vi "MoveRel.vi"(0 "ASI stage":T1, 1 "Axis configuration":u16(ring)=5 items=["No axis", "X", "Y", "Z", "XY", "XYZ"], 5 "x":dbl, 7 "y":dbl, 9 "z":dbl, 11 "error in (no error)":errorcluster) -> (4 "ASI stage out":T1, 15 "error out":errorcluster)   [LabVIEW 2010]
uses:
  stage properties.ctl
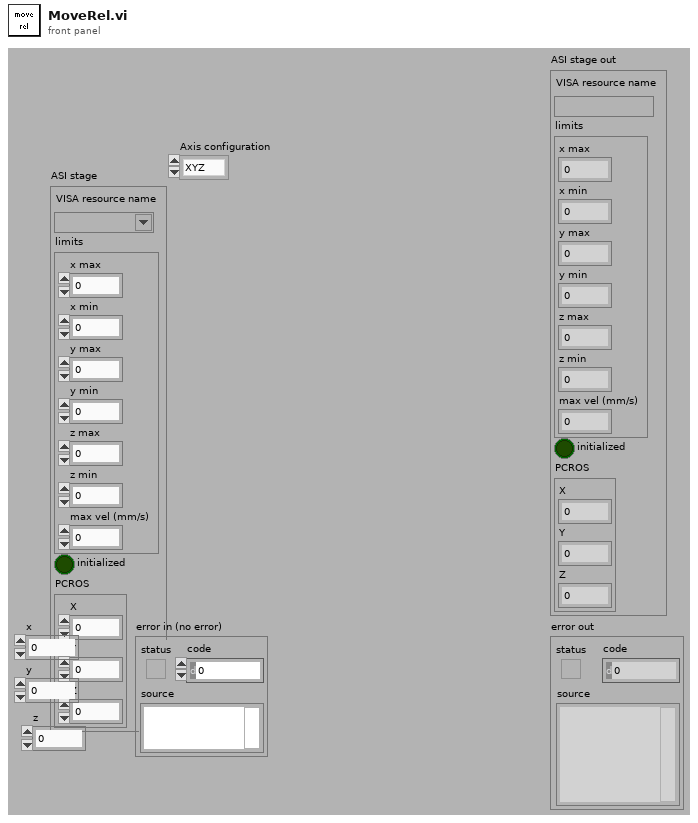
[diagram p1: front panel]
types:
  T1 = typedef "stage properties.ctl" = cluster{"VISA resource name":refnum<visa-resource-name>, "limits":cluster{"x max":dbl, "x min":dbl, "y max":dbl, "y min":dbl, "z max":dbl, "z min":dbl, "max vel (mm/s)":dbl}, "initialized":bool, "PCROS":cluster{"X":dbl, "Y":dbl, "Z":dbl}}
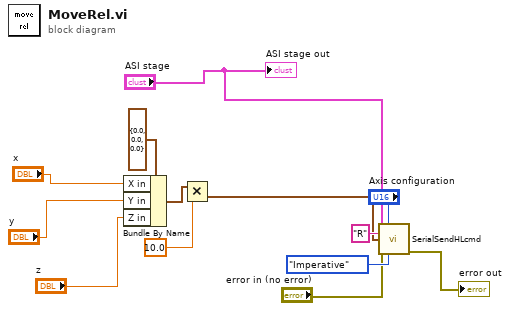
[diagram p0: block diagram]
diagram:
  n1 = Bundle By Name(cluster=cluster{"X in":dbl, "Y in":dbl, "Z in":dbl} {"X in"=0.0, "Y in"=0.0, "Z in"=0.0} ("data in"), "X in"="x", "Y in"="y", "Z in"="z") -> (w2:cluster{"X in":dbl, "Y in":dbl, "Z in":dbl})
  n2 = Multiply(x=w2, y=10.0 ("z")) -> (x*y=w3:cluster{"X in":dbl, "Y in":dbl, "Z in":dbl})
  n3 = call "SerialSendHLcmd.vi"("ASI stage"="ASI stage", "Axis configuration"="Axis configuration", "Command"="R", "data in"=w3, "error in (no error)"="error in (no error)", "Command type"=enum16{"Query", "Where", "Imperative", "DU Y"}."Imperative") -> ("error out"=→"error out":errorcluster)  [unwired: 7 in, 2 out]
  "ASI stage out" <- "ASI stage"
